vi "Set All.vi"(8 "error in (no error)":errorcluster, 9 "Camera Settings":T1={"Exposure Time (ms)"=100.0, "Binning"=enum."2x2", "Scan Mode"=-1, "Frames to Acquire"=1000.0, "Pixel Correction"=FALSE, "Frames to Skip"=1, "File Path"=path "", "Duty cycle"=1.0, "ALEX"=FALSE, "Shutter Enable"=[]} {"Exposure Time (ms)" min=1.0 max=10000.0 step=1.0}, 10 "Streaming?":bool, 11 "Synchronization Device in":refnum<class "Synchronization Device.lvclass">) -> (0 "error out":errorcluster, 3 "Synchronization Device out":refnum<class "Synchronization Device.lvclass">)   [LabVIEW 2018, in "Synchronization Device.lvlib" / "Synchronization Device.lvclass"]
uses:
  Synchronization Device.lvclass
  Resources/Type Defs/Camera Settings.ctl
  Synchronization Device.lvclass/Synchronization Device.ctl
  Resources/GLOBAL/GLOBAL Experiment Metadata.vi
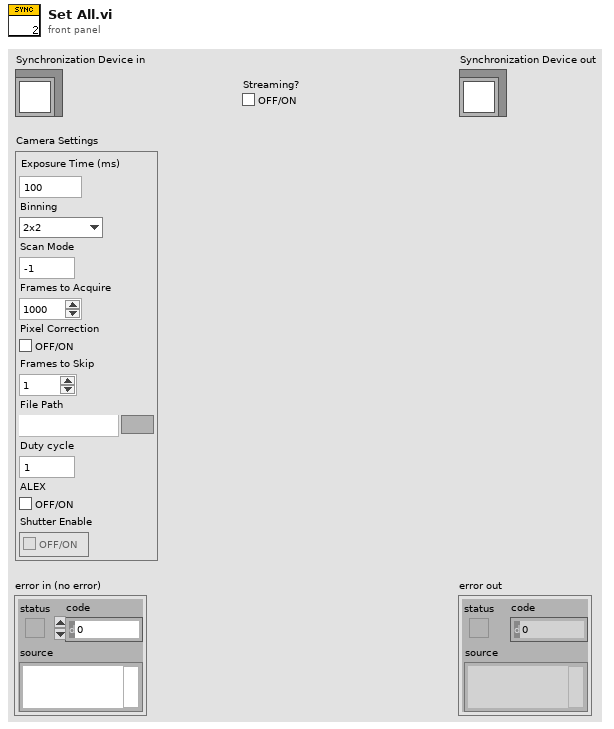
[diagram p1: front panel]
types:
  T1 = typedef "Camera Settings.ctl" = cluster{"Exposure Time (ms)":dbl, "Binning":enum16{"1x1", "2x2", "4x4"}, "Scan Mode":i32, "Frames to Acquire":dbl, "Pixel Correction":bool, "Frames to Skip":u32, "File Path":path, "Duty cycle":dbl, "ALEX":bool, "Shutter Enable":bool[]}
  T2 = cluster{"Shutter Enable":bool[], "Duty Cycle":dbl, "Wavelengths":dbl[], "ALEX?":bool}
  T3 = cluster{"Interval (ms)":dbl, "ALEX":bool, "Shutter Enable":bool[], "Stream":bool, "Duty Cycle":dbl}
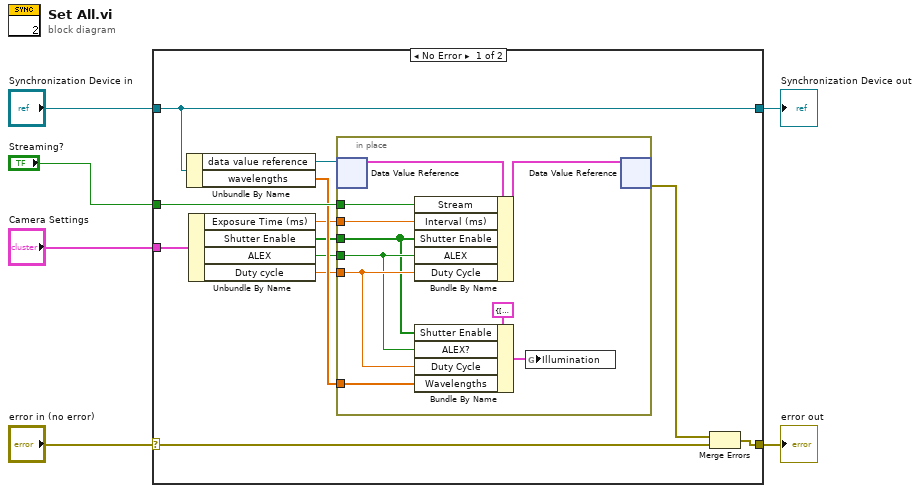
[diagram p0: block diagram]
diagram:
  n1 = case shown="No Error" "error in (no error)" {
    selector: "error in (no error)" -> [w16 w30]
    tunnel: [w17 w30] -> w5
    tunnel: [w18 w29] -> w3
    tunnel: "Synchronization Device in" -> [w18 w29]
    tunnel: "Streaming?" -> [w14 _]
    tunnel: "Camera Settings" -> [w11 _]
    frame No Error {
      n2 = Unbundle By Name(w18) -> ("data value reference"=w15:refnum<data-value>, "wavelengths"=w12:dbl[])
      n3 = Unbundle By Name(w11) -> ("Exposure Time (ms)"=w10:dbl, "Shutter Enable"=w9:bool[], "ALEX"=w8:bool, "Duty cycle"=w7:dbl)
      n4 = in-place {
        in-place-border: w14 -> [w27]
        in-place-border: w12 -> [w23]
        in-place-border: w10 -> [w22]
        in-place-border: w7 -> [w21]
        in-place-border: w8 -> [w20]
        in-place-border: w9 -> [w19]
        n5 = in-place-dvr #1(w15) -> (w26:T3)  [unwired: 1 out]
        n6 = Bundle By Name(cluster=w26, "Stream"=w27, "Interval (ms)"=w22, "Shutter Enable"=w19, "ALEX"=w20, "Duty Cycle"=w21) -> (w28:T3)
        n7 = Bundle By Name(cluster=T2 {"Shutter Enable"=[], "Duty Cycle"=0.0, "Wavelengths"=[], "ALEX?"=FALSE} ("Cluster"), "Shutter Enable"=w19, "ALEX?"=w20, "Duty Cycle"=w21, "Wavelengths"=w23) -> (w25:T2)
        n8 = global write "GLOBAL Experiment Metadata.vi" "Illumination"(w25) -> ()
        n9 = in-place-dvr #1(w28) -> (w13:errorcluster)  [unwired: 1 out]
      }
      n10 = Merge Errors(w13, w16) -> (w17:errorcluster)
    }
    frame Error {
    }
  }
  "error out" <- w5
  "Synchronization Device out" <- w3
